vi "SpinnerSecondMotorValue.vi"() -> ()   [LabVIEW 2016]
panel:
  out "SpinnerSecondMotorValue":dbl
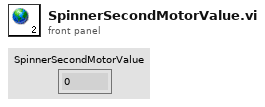
[diagram p1: front panel]
diagram:
